vi "SMO.UI.Example.SetDependencies.vi"(8 "error in (no error)":errorcluster, 10 "Dependencies":T1, 11 "SMO UI.Template in":refnum<class "SMO.UI.Example.lvclass">) -> (0 "error out":errorcluster, 3 "SMO UI.Template out":refnum<class "SMO.UI.Example.lvclass">)   [LabVIEW 2013, in "SMO.UI.Example.lvclass"]
uses:
  SMO.UI.Example.lvclass
  Typedefs/Dependencies--Cluster.ctl
  SMO.Example/SMO.Example.lvclass
  SMO.UI.Example.lvclass/SMO.UI.Example.ctl
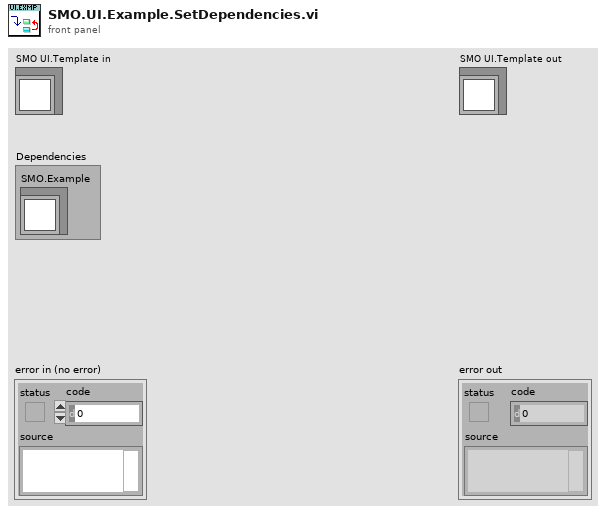
[diagram p1: front panel]
types:
  T1 = typedef "SMO.UI.Example.lvclass/Dependencies--Cluster.ctl" = cluster{"SMO.Example":refnum<class "SMO.Example.lvclass">}
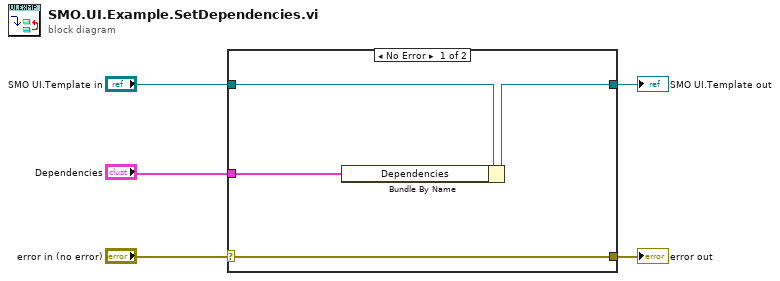
[diagram p0: block diagram]
diagram:
  n1 = case shown="No Error" "error in (no error)" {
    selector: "error in (no error)" -> [w9 w10]
    tunnel: [w9 w10] -> w4
    tunnel: [w7 w11] -> w2
    tunnel: "SMO UI.Template in" -> [w8 w11]
    tunnel: "Dependencies" -> [w6 _]
    frame No Error {
      n2 = Bundle By Name(cluster=w8, "Dependencies"=w6) -> (w7:refnum<class "SMO.UI.Example.lvclass">)
    }
    frame Error {
    }
  }
  "error out" <- w4
  "SMO UI.Template out" <- w2
